vi "Create Bulk CSV String.vi"(8 "Error In":errorcluster, 10 "Messages":T1[](array[typedef]), 11 "Bulk CSV Buffer In":string) -> (0 "Error Out":errorcluster, 2 "CSV Length":i32, 3 "Bulk CSV Buffer Out":string)   [LabVIEW 2017, in "Logger.lvlib" / "File.lvlib"]
uses:
  File.lvlib
  Public/Controls/Statement.ctl
  Public/Controls/Tag.ctl
  <vilib>/dlg_ctls.llb/Space Constant.vi
  <vilib>/Utility/error.llb/Trim Whitespace.vi
  Logger.lvlib
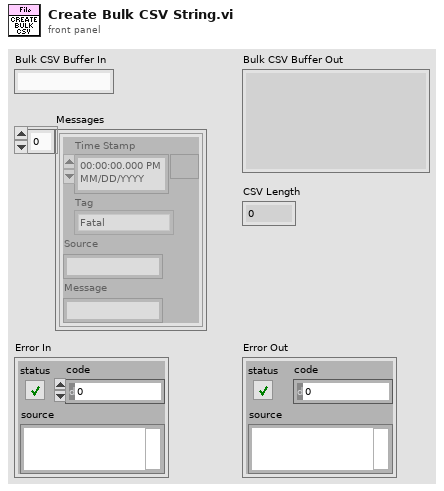
[diagram p1: front panel]
types:
  T1 = typedef "Logger.lvlib/Statement.ctl" = cluster{"Time Stamp":timestamp, "Tag":T2, "Source":string, "Message":string}
  T2 = typedef "Logger.lvlib/Tag.ctl" = enum16{"Fatal", "Error", "Warn", "Info", "Debug", "Trace"}
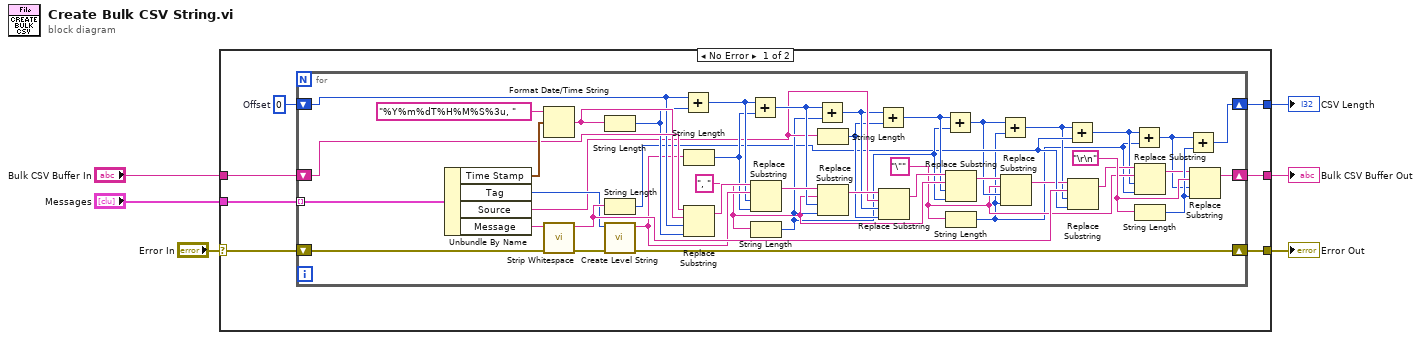
[diagram p0: block diagram]
diagram:
  n1 = case shown="No Error" "Error In" {
    selector: "Error In" -> [w13 w56]
    tunnel: [w12 w56] -> w5
    tunnel: "Messages" -> [w11 _]
    tunnel: "Bulk CSV Buffer In" -> [w10 _]
    tunnel: [w8 _] -> w2
    tunnel: [w7 _] -> w1
    frame No Error {
      w9 = 0  # Offset
      n2 = for {
        tunnel: w11 -> [w55] mode=indexing
        shift-right: [w25] -> w8
        shift-left: w10 -> [w46]
        shift-right: [w49] -> w12
        shift-left: w13 -> [w52]
        shift-right: [w24] -> w7
        shift-left: w9 -> [w44]
        w17 = "\""
        w27 = "\r\n"
        w31 = ", " ("substring (\"\")")
        n3 = Unbundle By Name(w55) -> ("Time Stamp"=w48:timestamp, "Tag"=w50:T2, "Source"=w35:string, "Message"=w54:string)
        n4 = Format Date/Time String(time format string (%c)="%Y%m%dT%H%M%S%3u, ", seconds (now)=w48) -> (date/time string=w45:string)  [unwired: 1 in]
        n5 = call "Strip Whitespace.vi"("Error In"=w52, "Text"=w54) -> ("Error Out"=w51:errorcluster, "Stripped Text"=w53:string)  [unwired: 8 in]
        n6 = String Length(string=w45) -> (length=w42:i32)
        n7 = String Length(string=w53) -> (length=w28:i32)
        n8 = call "Create Level String.vi"("Error In"=w51, "Level"=w50) -> ("Error Out"=w49:errorcluster, "String"=w41:string)  [unwired: 8 in]
        n9 = Add(x=w44, y=w42) -> (x+y=w40:i32)
        n10 = String Length(string=w41) -> (length=w39:i32)
        n11 = Replace Substring(2:w42, 3:w44, 4:w45, 5:w46) -> (1:w43:string)  [unwired: 1 out]
        n12 = Add(x=w40, y=w39) -> (x+y=w37:i32)
        n13 = Replace Substring(2:w39, 3:w40, 4:w41, 5:w43) -> (1:w38:string)  [unwired: 1 out]
        n14 = String Length(string=w31) -> (length=w29:i32)
        n15 = Add(x=w37, y=w29) -> (x+y=w34:i32)
        n16 = String Length(string=w35) -> (length=w33:i32)
        n17 = Replace Substring(2:w29, 3:w37, 4:w31, 5:w38) -> (1:w36:string)  [unwired: 1 out]
        n18 = Add(x=w34, y=w33) -> (x+y=w30:i32)
        n19 = Replace Substring(2:w33, 3:w34, 4:w35, 5:w36) -> (1:w32:string)  [unwired: 1 out]
        n20 = Add(x=w30, y=w29) -> (x+y=w21:i32)
        n21 = Replace Substring(2:w29, 3:w30, 4:w31, 5:w32) -> (1:w23:string)  [unwired: 1 out]
        n22 = String Length(string=w17) -> (length=w15:i32)
        n23 = Add(x=w21, y=w15) -> (x+y=w20:i32)
        n24 = Replace Substring(2:w15, 3:w21, 4:w17, 5:w23) -> (1:w22:string)  [unwired: 1 out]
        n25 = Add(x=w20, y=w28) -> (x+y=w16:i32)
        n26 = Replace Substring(2:w28, 3:w20, 4:w53, 5:w22) -> (1:w19:string)  [unwired: 1 out]
        n27 = Add(x=w16, y=w15) -> (x+y=w14:i32)
        n28 = Replace Substring(2:w15, 3:w16, 4:w17, 5:w19) -> (1:w18:string)  [unwired: 1 out]
        n29 = String Length(string=w27) -> (length=w26:i32)
        n30 = Add(x=w14, y=w26) -> (x+y=w24:i32)
        n31 = Replace Substring(2:w26, 3:w14, 4:w27, 5:w18) -> (1:w25:string)  [unwired: 1 out]
      }
    }
    frame Error {
    }
  }
  "Error Out" <- w5
  "Bulk CSV Buffer Out" <- w2
  "CSV Length" <- w1
